vi "GetTargetName.vi"(8 "error in (no error)":errorcluster, 11 "VIA in":refnum<class "VIA.lvclass">) -> (0 "error out":errorcluster, 2 "TargetName":string, 3 "VIA out":refnum<class "VIA.lvclass">)   [LabVIEW 2012, in "VIA.lvclass"]
uses:
  <vilib>/NXT/LegoClasses/VIA/VIA.lvclass
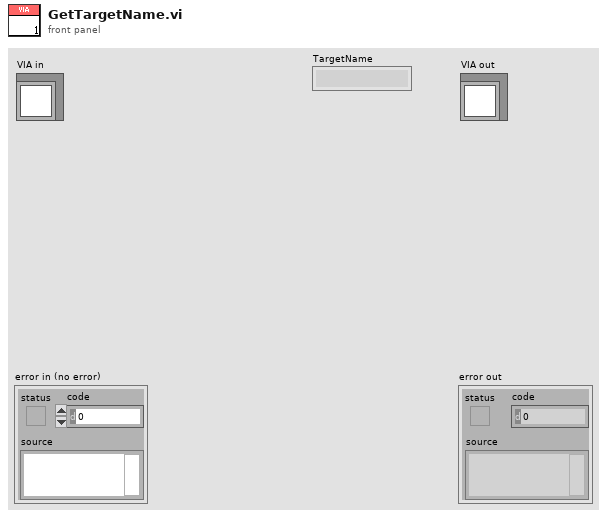
[diagram p1: front panel]
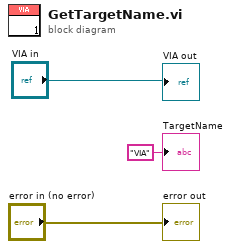
[diagram p0: block diagram]
diagram:
  "error out" <- "error in (no error)"
  "VIA out" <- "VIA in"
  "TargetName" <- "VIA" ("TargetName")
